vi "MotorInit.vi"(8 "error in":errorcluster) -> (0 "error out":errorcluster)   [LabVIEW 2014]
uses:
  <vilib>/Rock Robotics/WPI/CAN/TalonSRX/WPI_CANTalonSRX_APIFeedbackSelect.ctl
  <vilib>/Rock Robotics/WPI/CAN/TalonSRX/WPI_CANTalonSRX_APIControlMode.ctl
panel:
  out "Encoder Velocity":dbl
  in  "Gantry PID Gains":T1={"proportional gain (Kc)"=3.0, "integral time (Ti, min)"=0.0, "derivative time (Td, min)"=1.0}
  in  "Lift PID Gains":T1={"proportional gain (Kc)"=65.0, "integral time (Ti, min)"=0.0, "derivative time (Td, min)"=35.0}
  # "P=4, d=1.2"
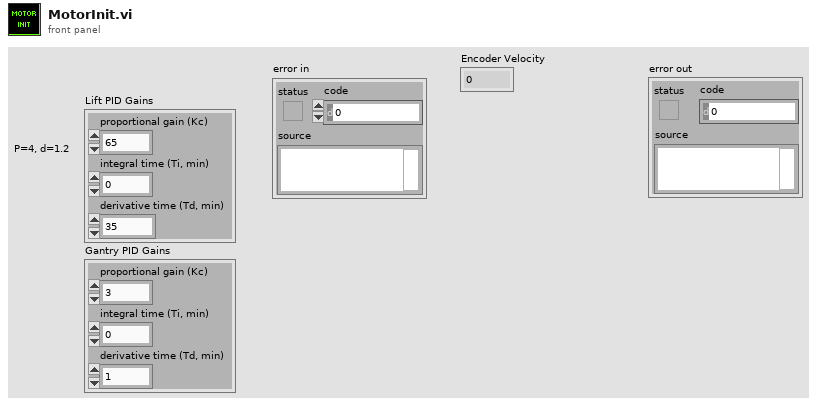
[diagram p1: front panel]
types:
  T1 = cluster{"proportional gain (Kc)":dbl, "integral time (Ti, min)":dbl, "derivative time (Td, min)":dbl}
  T2 = typedef "WPI_CANTalonSRX_APIControlMode.ctl" = enum8{"Percent VBus", "Speed", "Position", "Slave", "Unchanged / Invalid"}
  T3 = typedef "WPI_CANTalonSRX_APIFeedbackSelect.ctl" = enum16{"Digital Quadrature Encoder", "Analog Potentiometer", "Analog Encoder"}
  T4 = typedef "WPI_MotorControlDeviceRef.ctl" = cluster{"DeviceStatus":errorcluster, "Type":T5, "PWM":cluster{"Controller":T6, "PWM Channel":T7, "DeadBand":T8}, "CAN":cluster{"Device Number":u8, "Control Mode":T9, "Semaphore":T10, "Max Vout":dbl, "TalonSRX Control Mode":T2}, "Invert":bool, "TransformRef":T11, "InvTransformRef":T11}
  T5 = typedef "WPI_MotorControlType.ctl" = enum16{"PWM", "CAN", "CANTalonSRX"}
  T6 = typedef "FPGA_TypedefDigitalModule.ctl" = enum16{"Controller 1"}
  T7 = typedef "FPGA_DIOPWMChannel.ctl" = enum8{"PWM 0", "PWM 1", "PWM 2", "PWM 3", "PWM 4", "PWM 5", "PWM 6", "PWM 7", "PWM 8", "PWM 9", "PWM MXP 0", "PWM MXP 1", "PWM MXP 2", "PWM MXP 3", "PWM MXP 4", "PWM MXP 5", "PWM MXP 6", "PWM MXP 7", "PWM MXP 8", "PWM MXP 9", "Invalid"}
  T8 = typedef "WPI_PWMDeadband.ctl" = cluster{"Name":string, "maxPositivePwm":i32, "minPositivePwm":i32, "centerPwm":i32, "maxNegativePwm":i32, "minNegativePwm":i32, "angularRange":u16}
  T9 = typedef "WPI_CANJaguar_ControlMode.ctl" = enum8{"Percent VBus", "Current", "Speed", "Position", "Voltage"}
  T10 = typedef "Semaphore RefNum" = refnum<k1>
  T11 = typedef "WPI_PWMTransform_ConPane.ctl" = refnum<vi>
  T12 = typedef "WPI_CANTalonSRX_GlobalStatus.ctl" = cluster{"Applied Throttle":dbl, "Module Enabled":bool, "CAN Error":errorcluster, "Closed Loop Error":dbl, "Forward Limit Switch Closed":bool, "Reverse Limit Switch Closed":bool, "Sensor Position":dbl, "Sensor Velocity":dbl, "Current":dbl, "Sticky Fault - Over Temp":bool, "Sticky Fault - Under Voltage":bool, "Sticky Fault - Forward Limit":bool, "Sticky Fault - Reverse Limit":bool, "Sticky Fault - Forward Soft Limit":bool, "Sticky Fault - Reverse Soft Limit":bool, "Brake is Enabled":bool, "Encoder Position":dbl, "Encoder Velocity":dbl, "Encoder Index Count":dbl, "Encoder A Pin State":bool, "Encoder B Pin State":bool, "Encoder Index Pin State":bool, "Analog In":dbl, "Analog In Velocity":dbl, "Temperature (C)":dbl, "Battery Voltage":dbl}
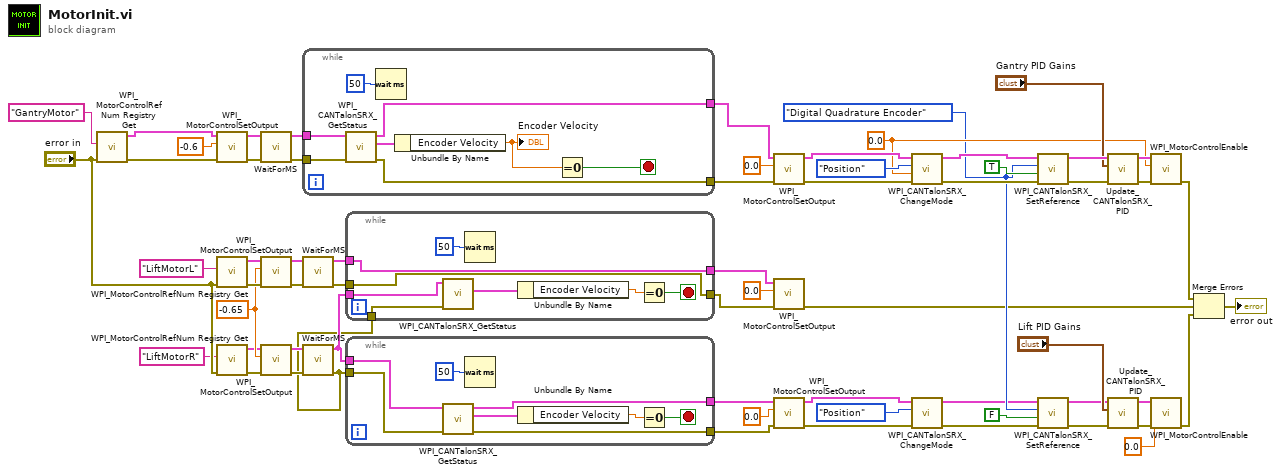
[diagram p0: block diagram]
diagram:
  w31 = -0.65 ("Output")
  w36 = WPI_CANTalonSRX_APIFeedbackSelect."Digital Quadrature Encoder" ("Feedback Reference")
  w38 = 0.0 ("Output")
  n1 = call <vilib>:"WPI_MotorControlRefNum Registry Get.vi"("error in (no error)"="error in", "refnum name"="GantryMotor") -> ("error out"=w60:errorcluster, "MotorControlDevRef"=w59:T4)  [unwired: 8 in]
  n2 = call <vilib>:"WPI_MotorControlSetOutput.vi"("error in (no error)"=w60, "Output"=-0.6, "MotorControlDevRef"=w59) -> ("error out"=w50:errorcluster, "MotorControlDevRef"=w51:T4)  [unwired: 6 in, 1 out]
  n3 = call <vilib>:"WPI_MotorControlRefNum Registry Get.vi"("error in (no error)"="error in", "refnum name"="LiftMotorL") -> ("error out"=w34:errorcluster, "MotorControlDevRef"=w33:T4)  [unwired: 8 in]
  n4 = call <vilib>:"WPI_MotorControlRefNum Registry Get.vi"("error in (no error)"="error in", "refnum name"="LiftMotorR") -> ("error out"=w25:errorcluster, "MotorControlDevRef"=w24:T4)  [unwired: 8 in]
  n5 = call "WaitForMS.vi"("error in"=w50, "MotorControlDevRef"=w51) -> ("error out"=w48:errorcluster, "MotorControlDevRef 2"=w49:T4)  [unwired: 8 in]
  n6 = call <vilib>:"WPI_MotorControlSetOutput.vi"("error in (no error)"=w34, "Output"=w31, "MotorControlDevRef"=w33) -> ("error out"=w28:errorcluster, "MotorControlDevRef"=w29:T4)  [unwired: 6 in, 1 out]
  n7 = call <vilib>:"WPI_MotorControlSetOutput.vi"("error in (no error)"=w25, "Output"=w31, "MotorControlDevRef"=w24) -> ("error out"=w8:errorcluster, "MotorControlDevRef"=w9:T4)  [unwired: 6 in, 1 out]
  n8 = while {
    tunnel: w49 -> [w69]
    tunnel: w48 -> [w68]
    tunnel: [w65] -> w54
    tunnel: [w64] -> w53
    stop <- w63 stop-if-true
    n9 = call <vilib>:"WPI_CANTalonSRX_GetStatus.vi"("error in (no error)"=w68, "CAN Talon SRX Ref"=w69) -> ("error out"=w64:errorcluster, "Talon SRX Status"=w67:T12, "CAN Talon SRX Ref Out"=w65:T4)  [unwired: 7 in]
    n10 = Wait (ms)(milliseconds to wait=u32 50) -> ()  [unwired: 1 out]
    n11 = Unbundle By Name(w67) -> ("Encoder Velocity"=w66:dbl)
    "Encoder Velocity" <- w66
    n12 = Equal To 0?(x=w66) -> (x = 0?=w63:bool)
  }
  n13 = call "WaitForMS.vi"("error in"=w28, "MotorControlDevRef"=w29) -> ("error out"=w27:errorcluster, "MotorControlDevRef 2"=w26:T4)  [unwired: 8 in]
  n14 = call "WaitForMS.vi"("error in"=w8, "MotorControlDevRef"=w9) -> ("error out"=w6:errorcluster, "MotorControlDevRef 2"=w7:T4)  [unwired: 8 in]
  n15 = while {
    tunnel: w26 -> [w72]
    tunnel: w27 -> [w71]
    tunnel: w7 -> [w74]
    tunnel: w6 -> [w73]
    tunnel: [w72] -> w5
    tunnel: [w71] -> w4
    stop <- w75 stop-if-true
    n16 = call <vilib>:"WPI_CANTalonSRX_GetStatus.vi"("error in (no error)"=w73, "CAN Talon SRX Ref"=w74) -> ("Talon SRX Status"=w77:T12)  [unwired: 7 in, 2 out]
    n17 = Wait (ms)(milliseconds to wait=u32 50) -> ()  [unwired: 1 out]
    n18 = Unbundle By Name(w77) -> ("Encoder Velocity"=w76:dbl)
    n19 = Equal To 0?(x=w76) -> (x = 0?=w75:bool)
  }
  n20 = while {
    tunnel: w7 -> [w85]
    tunnel: w6 -> [w84]
    tunnel: [w81] -> w11
    tunnel: [w80] -> w10
    stop <- w79 stop-if-true
    n21 = call <vilib>:"WPI_CANTalonSRX_GetStatus.vi"("error in (no error)"=w84, "CAN Talon SRX Ref"=w85) -> ("error out"=w80:errorcluster, "Talon SRX Status"=w83:T12, "CAN Talon SRX Ref Out"=w81:T4)  [unwired: 7 in]
    n22 = Wait (ms)(milliseconds to wait=u32 50) -> ()  [unwired: 1 out]
    n23 = Unbundle By Name(w83) -> ("Encoder Velocity"=w82:dbl)
    n24 = Equal To 0?(x=w82) -> (x = 0?=w79:bool)
  }
  n25 = call <vilib>:"WPI_MotorControlSetOutput.vi"("error in (no error)"=w53, "Output"=0.0, "MotorControlDevRef"=w54) -> ("error out"=w55:errorcluster, "MotorControlDevRef"=w56:T4)  [unwired: 6 in, 1 out]
  n26 = call <vilib>:"WPI_MotorControlSetOutput.vi"("error in (no error)"=w4, "Output"=0.0, "MotorControlDevRef"=w5) -> ("error out"=w2:errorcluster)  [unwired: 6 in, 2 out]
  n27 = call <vilib>:"WPI_MotorControlSetOutput.vi"("error in (no error)"=w10, "Output"=0.0, "MotorControlDevRef"=w11) -> ("error out"=w19:errorcluster, "MotorControlDevRef"=w20:T4)  [unwired: 6 in, 1 out]
  n28 = call <vilib>:"WPI_CANTalonSRX_ChangeMode.vi"("error in (no error)"=w55, "Output"=w38, "Control Mode"=WPI_CANTalonSRX_APIControlMode."Position", "CAN Talon SRX Ref"=w56) -> ("error out"=w44:errorcluster, "CAN Talon SRX Ref Out"=w43:T4)  [unwired: 6 in]
  n29 = call <vilib>:"WPI_CANTalonSRX_ChangeMode.vi"("error in (no error)"=w19, "Control Mode"=WPI_CANTalonSRX_APIControlMode."Position", "CAN Talon SRX Ref"=w20) -> ("error out"=w16:errorcluster, "CAN Talon SRX Ref Out"=w15:T4)  [unwired: 7 in]
  n30 = call <vilib>:"WPI_CANTalonSRX_SetReference.vi"("error in (no error)"=w44, "Reverse Feedback Sensor"=TRUE, "Feedback Reference"=w36, "CAN Talon SRX Ref"=w43) -> ("error out"=w41:errorcluster, "CAN Talon SRX Ref Out"=w42:T4)  [unwired: 6 in]
  n31 = call <vilib>:"WPI_CANTalonSRX_SetReference.vi"("error in (no error)"=w16, "Reverse Feedback Sensor"=FALSE, "Feedback Reference"=w36, "CAN Talon SRX Ref"=w15) -> ("error out"=w13:errorcluster, "CAN Talon SRX Ref Out"=w14:T4)  [unwired: 6 in]
  n32 = call "Update_CANTalonSRX_PID.vi"("error in (no error)"=w41, "PID Gains"="Gantry PID Gains", "CAN Talon SRX Ref"=w42) -> ("error out"=w45:errorcluster, "CAN Talon SRX Ref Out"=w46:T4)  [unwired: 7 in]
  n33 = call "Update_CANTalonSRX_PID.vi"("error in (no error)"=w13, "PID Gains"="Lift PID Gains", "CAN Talon SRX Ref"=w14) -> ("error out"=w17:errorcluster, "CAN Talon SRX Ref Out"=w18:T4)  [unwired: 7 in]
  n34 = call <vilib>:"WPI_MotorControlEnable.vi"("error in (no error)"=w45, "Encoder Initial Position"=w38, "CAN Jaguar Ref"=w46) -> ("error out"=w62:errorcluster)  [unwired: 7 in, 1 out]
  n35 = call <vilib>:"WPI_MotorControlEnable.vi"("error in (no error)"=w17, "Encoder Initial Position"=0.0, "CAN Jaguar Ref"=w18) -> ("error out"=w61:errorcluster)  [unwired: 7 in, 1 out]
  n36 = Merge Errors(w62, w2, w61) -> (→"error out":errorcluster)
